vi "griper.vi"   [LabVIEW 2015]
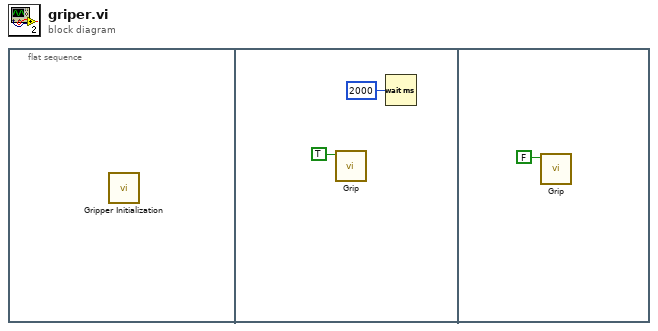
[diagram p0: block diagram]
diagram:
  n1 = flat-sequence {
    frame #0 {
      n2 = call "Gripper Initialization.vi"() -> ()  [unwired: 12 in]
    }
    frame #1 {
      n3 = call "Grip.vi"("Grip"=TRUE) -> ()  [unwired: 11 in]
      n4 = Wait (ms)(milliseconds to wait=u32 2000) -> ()  [unwired: 1 out]
    }
    frame #2 {
      n5 = call "Grip.vi"("Grip"=FALSE) -> ()  [unwired: 11 in]
    }
  }
